vi "ReadTemperature.vi"(8 "error in (no error)":errorcluster, 11 "VISA Refnum in":refnum<visa-resource-name>) -> (0 "error in (no error) 2":errorcluster, 1 "Temperature (°C)":dbl, 2 "read buffer":string, 3 "VISA Refnum Out":refnum<visa-resource-name>)   [LabVIEW 2023]
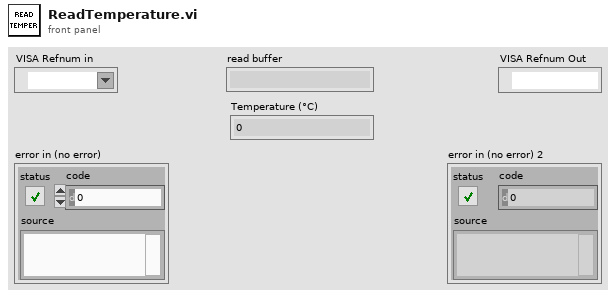
[diagram p1: front panel]
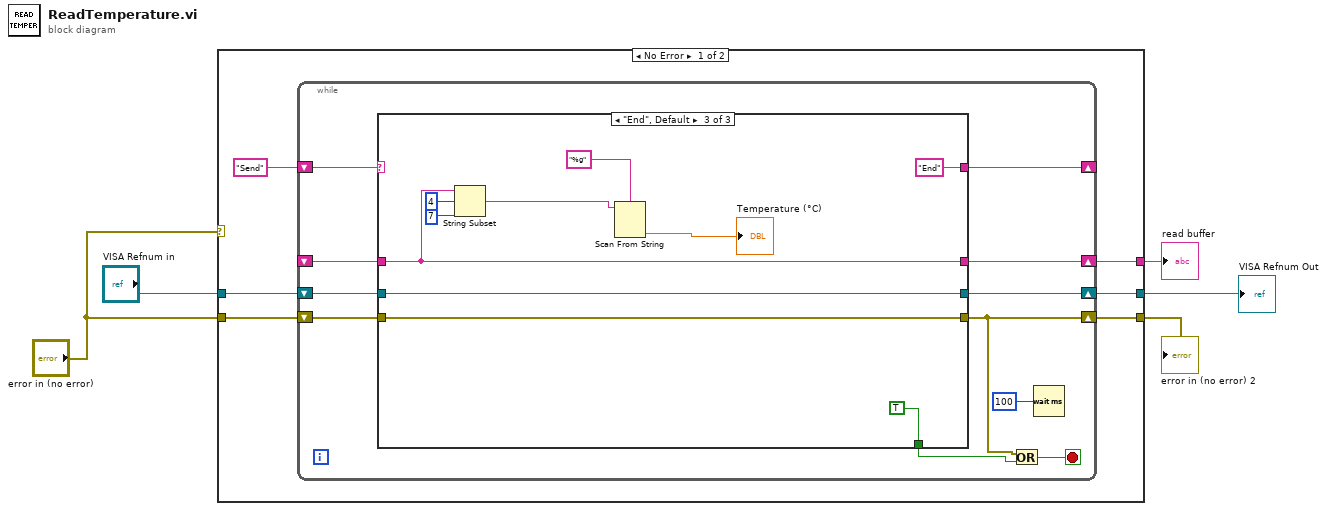
[diagram p0: block diagram]
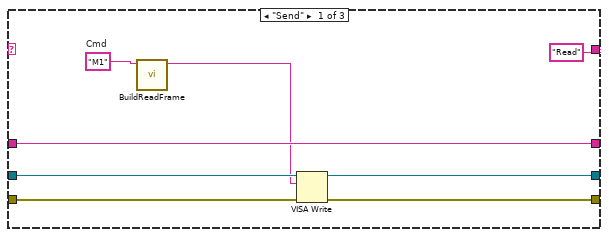
[diagram p2: hidden frame]
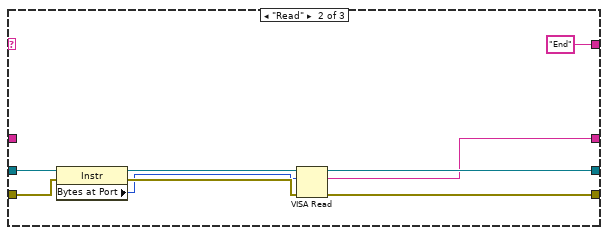
[diagram p3: hidden frame]
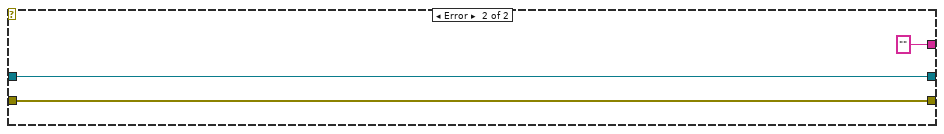
[diagram p4: hidden frame]
diagram:
  n1 = case shown="No Error" "error in (no error)" {
    tunnel: "VISA Refnum in" -> [w11 w51]
    tunnel: "error in (no error)" -> [w10 w50]
    tunnel: [w8 "" ("read buffer")] -> w3
    tunnel: [w7 w51] -> w1
    tunnel: [w6 w50] -> w2
    frame No Error {
      n2 = while {
        shift-right: [w19] -> _
        shift-left: "Send" -> [w20]
        shift-right: [w14] -> w7
        shift-left: w11 -> [w22]
        shift-right: [w15] -> w6
        shift-left: w10 -> [w21]
        shift-right: [w13] -> w8
        shift-left: _ -> [w12]
        stop <- w17 stop-if-true
        n3 = case shown="\"End\", Default" w20 {
          tunnel: w22 -> [w29 w39 w47]
          tunnel: w21 -> [w28 w38 w48]
          tunnel: ["Read" "End" "End"] -> w19
          tunnel: [_ _ TRUE] -> w16
          tunnel: [w26 w33 w48] -> w15
          tunnel: [w25 w34 w47] -> w14
          tunnel: [w24 w32 w45] -> w13
          tunnel: w12 -> [w24 _ w45]
          frame "Send" {
            w30 = "M1"  # Cmd
            n4 = call "BuildReadFrame.vi"("Cmd"=w30) -> ("String"=w23:string)  [unwired: 10 in]
            n5 = VISA Write(VISA resource name=w29, write buffer=w23, error in (no error)=w28) -> (VISA resource name out=w25:refnum<visa-resource-name>, error out=w26:errorcluster)  [unwired: 1 out]
          }
          frame "Read" {
            n6 = property class="Instr"(reference=w39, error in=w38) -> (reference out=w37:refnum<visa-resource-name>, error out=w36:errorcluster, "Bytes at Port"=w35:u32)
            n7 = VISA Read(VISA resource name=w37, byte count=w35, error in (no error)=w36) -> (VISA resource name out=w34:refnum<visa-resource-name>, read buffer=w32:string, error out=w33:errorcluster)  [unwired: 1 out]
          }
          frame "End", Default {
            n8 = String Subset(string=w45, offset (0)=4, length (rest)=7 ("length (rest)")) -> (substring=w42:string)
            n9 = Scan From String(format string="%g", input string=w42) -> (output 1=→"Temperature (°C)":dbl)  [unwired: 3 in, 3 out]
          }
        }
        n10 = Or(x=w15, y=w16) -> (x .or. y?=w17:bool)
        n11 = Wait (ms)(milliseconds to wait=u32 100) -> ()  [unwired: 1 out]
      }
    }
    frame Error {
    }
  }
  "read buffer" <- w3
  "VISA Refnum Out" <- w1
  "error in (no error) 2" <- w2
